vi "Git Examine Config.vi"() -> ()   [LabVIEW 2019, in "Git.lvclass"]
uses:
  Git.lvclass
  <vilib>/Utility/config.llb/Read Key (String).vi
  <vilib>/Utility/config.llb/NI_LVConfig.lvlib
panel:
  out "Contents":string
  out "Value":string
  out "Keys":i32(listbox)
  out "Sections":i32(listbox)
  in  "Repository Path":path=path "C:/Users/patrick/Documents/GitHub/Oxford-1820"
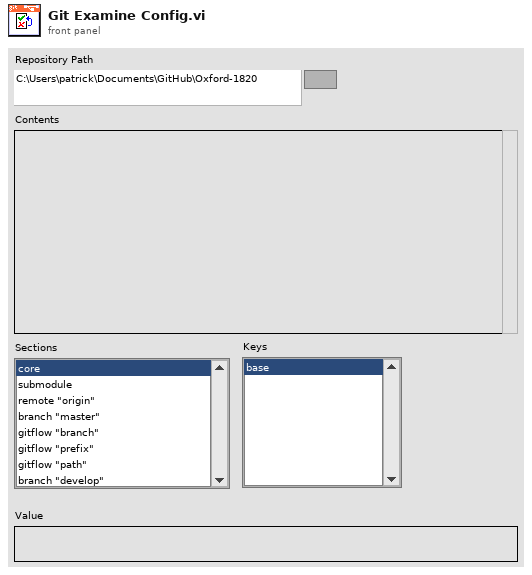
[diagram p1: front panel]
types:
  T1 = typedef "NI_LVConfig.lvlib/Config Data RefNum.ctl" = refnum<k1>
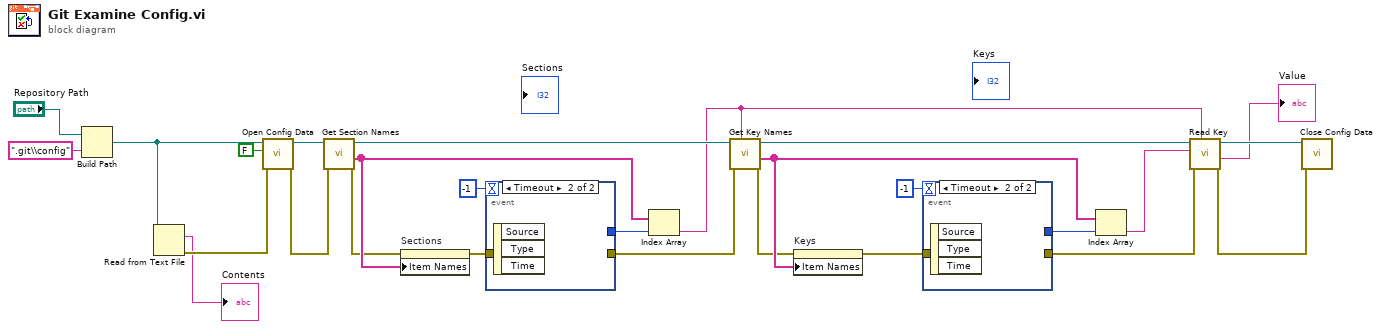
[diagram p0: block diagram]
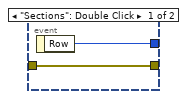
[diagram p2: hidden frame]
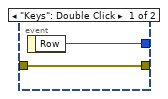
[diagram p3: hidden frame]
diagram:
  n1 = Build Path(base path="Repository Path", name or relative path=".git\\config") -> (appended path=w5:path)
  n2 = Read from Text File(file (use dialog)=w5) -> (text=→"Contents":string, error out=w4:errorcluster)  [unwired: 3 in, 2 out]
  n3 = call <vilib>:"Open Config Data.vi"("error in (no error)"=w4, "create file if necessary (T)"=FALSE, "configuration file path"=w5) -> ("error out"=w26:errorcluster, "refnum"=w27:T1)  [unwired: 6 in, 1 out]
  n4 = call <vilib>:"Get Section Names.vi"("error in (no error)"=w26, "refnum"=w27) -> ("error out"=w15:errorcluster, "section names"=w17:string[], "refnum out"=w24:T1)  [unwired: 7 in]
  n5 = property on="Sections" class="LstBox (strict)"(error in=w15, "Item Names"=w17) -> (error out=w19:errorcluster)  [unwired: 1 in, 1 out]
  n6 = event shown="[1] Timeout" {
    selector: _ -> [_ _]
    dyn-events: _ -> [_ _]
    timeout: -1 -> [_ _]
    tunnel: w19 -> [w28 _]
    tunnel: [w29 _] -> w18
    tunnel: [w28 _] -> w10
    event "Sections": Double Click {
      n7 = event-data() -> ("Row"=w29:i32)  [unwired: 1 in]
    }
    event Timeout {
      n8 = event-data() -> ()  [unwired: 1 in, 3 out]
    }
  }
  n9 = Index Array(array=w17, index=w18) -> (element=w16:string)
  n10 = call <vilib>:"Get Key Names.vi"("section"=w16, "error in (no error)"=w10, "refnum"=w24) -> ("error out"=w9:errorcluster, "key names"=w12:string[], "refnum out"=w23:T1)  [unwired: 5 in, 1 out]
  n11 = property on="Keys" class="LstBox (strict)"(error in=w9, "Item Names"=w12) -> (error out=w14:errorcluster)  [unwired: 1 in, 1 out]
  n12 = event shown="[1] Timeout" {
    selector: _ -> [_ _]
    dyn-events: _ -> [_ _]
    timeout: -1 -> [_ _]
    tunnel: w14 -> [w30 _]
    tunnel: [w31 _] -> w13
    tunnel: [w30 _] -> w8
    event "Keys": Double Click {
      n13 = event-data() -> ("Row"=w31:i32)  [unwired: 1 in]
    }
    event Timeout {
      n14 = event-data() -> ()  [unwired: 1 in, 3 out]
    }
  }
  n15 = Index Array(array=w12, index=w13) -> (element=w11:string)
  n16 = call-poly <vilib>:"Read Key.vi"("section"=w16, "error in (no error)"=w8, "key"=w11, "refnum"=w23) -> ("error out"=w22:errorcluster, "value"=→"Value":string, "refnum out"=w21:T1)  [unwired: 4 in, 1 out]
  n17 = call <vilib>:"Close Config Data.vi"("error in (no error)"=w22, "refnum"=w21) -> ()  [unwired: 8 in, 2 out]
